vi "Create.vi"(7 "mode settings":variant, 8 "error in":errorcluster, 9 "number of default channels":i32, 10 "channel settings":variant, 11 "digital input mode in":refnum<class "Digital Input Mode.lvclass">) -> (0 "error out":errorcluster, 1 "channels":refnum<class "Channel.lvclass">[](array[class]), 3 "digital input mode out":refnum<class "Digital Input Mode.lvclass">)   [LabVIEW 2017, in "Scan Engine Scripting.lvlib" / "Digital Input Mode.lvclass"]
uses:
  Digital Input Mode.lvclass
  Channel Classes/Channel/Channel.lvclass
  Controls/digital channel settings.ctl
  36675302-4af7-49e3-a190-4f3a07b1a691.vi
  Channel Classes/DI Channel/DI Channel.lvclass
  C:/Users/nitest/Documents/niveristand-scan-engine-ethercat-custom-device/Custom Device Source/Scripting/Modules/Channel Classes/Channel/Channel.lvclass
  Scan Engine Scripting.lvlib
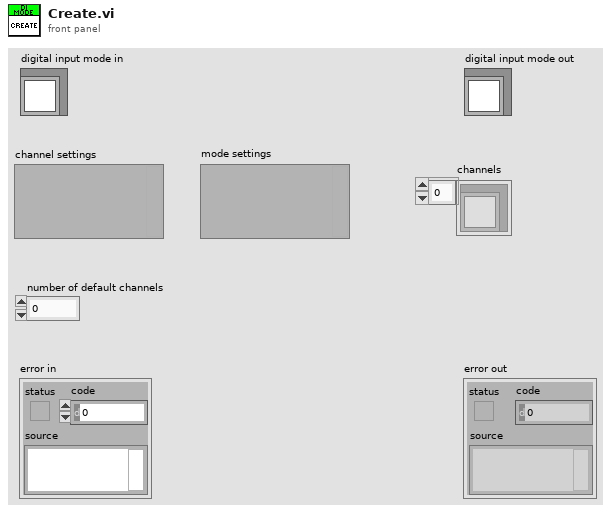
[diagram p1: front panel]
types:
  T1 = typedef "Scan Engine Scripting.lvlib/digital channel settings.ctl" = cluster{"name":string, "default value":bool}
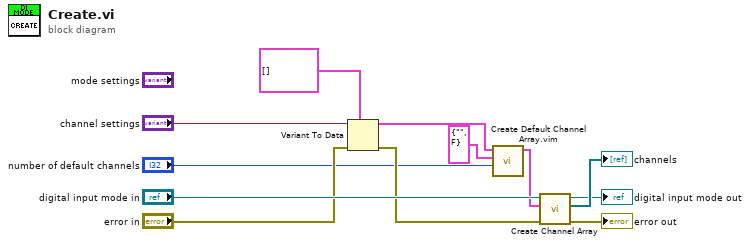
[diagram p0: block diagram]
diagram:
  n1 = Variant To Data(error in="error in", type=T1[] [] ("channel settings"), Variant="channel settings") -> (data=w3:T1[], error out=w6:errorcluster)
  n2 = call "Create Default Channel Array.vim"("number of default channels"="number of default channels", "default settings"=T1 {"name"="", "default value"=FALSE} ("channel settings"), "channel settings in"=w3) -> ("channel settings out"=w2:T1[])  [unwired: 8 in]
  n3 = call "Create Channel Array.vi"("error in"=w6, "channel settings"=w2, "digital input mode in"="digital input mode in") -> ("error out"=→"error out":errorcluster, "channels"=→"channels":refnum<class "DI Channel.lvclass">[], "digital input mode out"=→"digital input mode out":refnum<class "Digital Input Mode.lvclass">)  [unwired: 6 in]
